vi "monochromatorCommandGetBandpass.vi"(8 "error in":errorcluster, 11 "monochromator":refnum<k24>) -> (0 "error out":errorcluster, 2 "bandpass":dbl, 3 "monochromator":refnum<k24>)   [LabVIEW 2009]
doc: "Get Bandpass\nreturns double"
uses:
  C:/Users/anderson.chen/Desktop/Software Development/Cornerstone Series API (LV9)/Cornerstone DLL/Cornerstone.dll
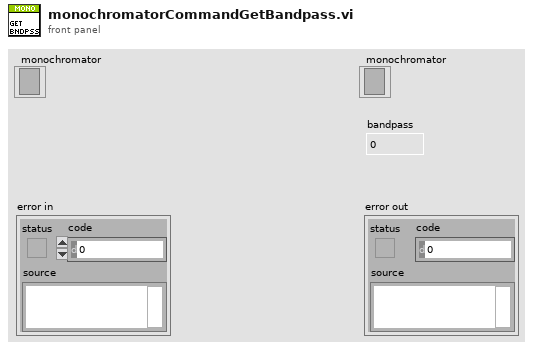
[diagram p1: front panel]
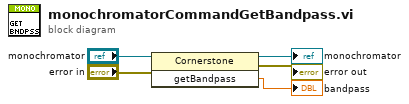
[diagram p0: block diagram]
diagram:
  n1 = invoke class="Cornerstone" method="getBandpass"(reference="monochromator", error in="error in") -> (reference out=→"monochromator":refnum<k24>, error out=→"error out":errorcluster, "getBandpass"=→"bandpass":dbl)  [unwired: 1 in]
